vi "Startup_LV2G-Paths.vi"(8 "error in (no error)":errorcluster, 10 "Paths":T1, 11 "Action":enum16{"Read", "Write"}(ring)=enum."Write") -> (0 "error out":errorcluster, 2 "Paths":T1)   [LabVIEW 2016]
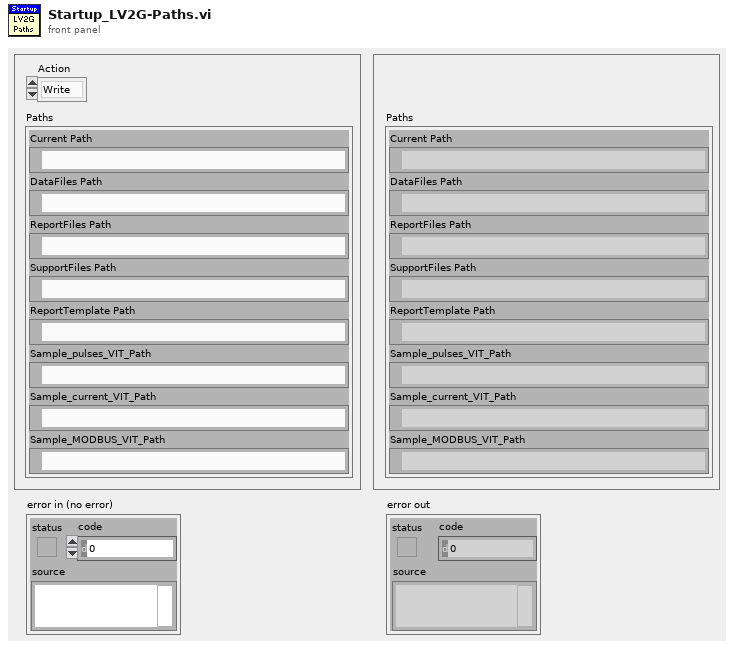
[diagram p1: front panel]
types:
  T1 = cluster{"Current Path":path, "DataFiles Path":path, "ReportFiles Path":path, "SupportFiles Path":path, "ReportTemplate Path":path, "Sample_pulses_VIT_Path":path, "Sample_current_VIT_Path":path, "Sample_MODBUS_VIT_Path":path}
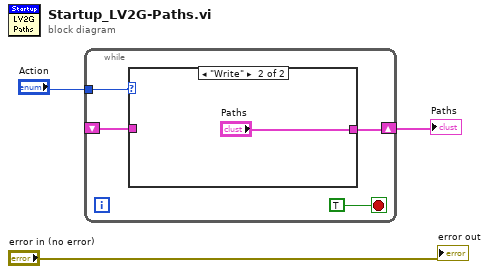
[diagram p0: block diagram]
diagram:
  n1 = while {
    tunnel: "Action" -> [w6]
    shift-right: [w5] -> w2
    shift-left: _ -> [w4]
    stop <- TRUE stop-if-true
    n2 = case shown="\"Write\"" w6 {
      tunnel: [w8 "Paths"] -> w5
      tunnel: w4 -> [w8 _]
      frame "Read", Default {
      }
      frame "Write" {
      }
    }
  }
  "Paths" <- w2
  "error out" <- "error in (no error)"
